vi "TrackStats2.vi"(0 "Last trial successful?":bool, 5 "Trial bin size":i32=100, 9 "Persistent\n Mode?":bool, 11 "Command":T1(ring)) -> (1 "Total incorrect":i32, 3 "Total correct":i32, 4 "# total trials":i32, 6 "Total % correct":dbl, 10 "Segment trials":i32, 12 "Experiment trials":i32, 13 "Experiment correct":i32, 14 "Experiment %":dbl, 15 "Segment Percentage":dbl)   [LabVIEW 2010]
panel:
  out "Experiment incorrect":i32
  out "Segment incorrect trials":i32
  out "Segment correct trials":i32
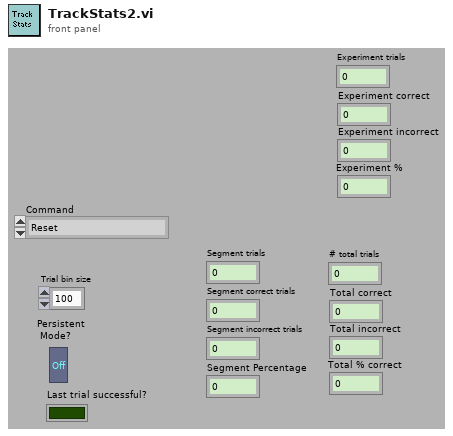
[diagram p1: front panel]
types:
  T1 = enum16{"Reset", "Increment", "Reset for exp", "Initialize"}
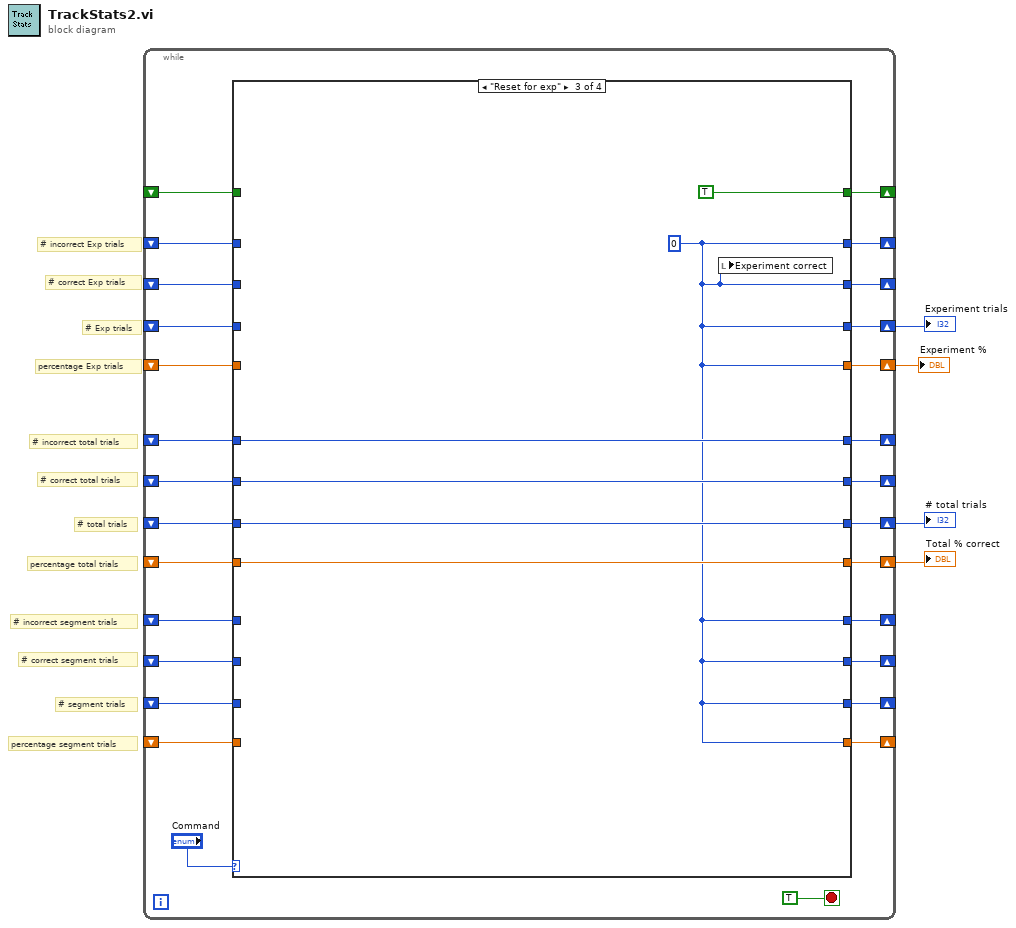
[diagram p0: block diagram]
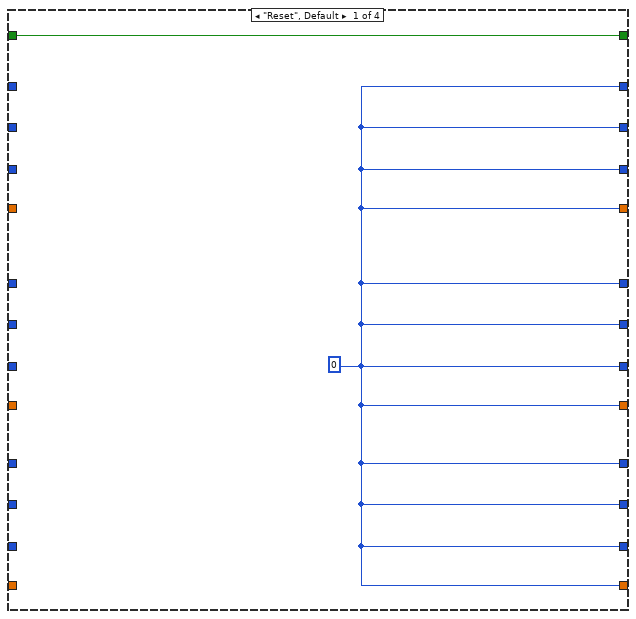
[diagram p2: hidden frame]
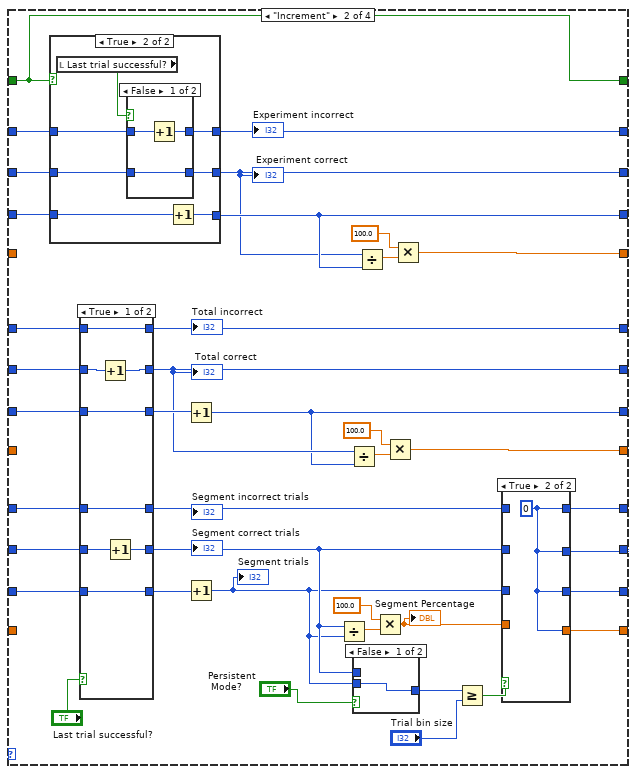
[diagram p3: hidden frame]
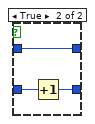
[diagram p5: hidden frame]
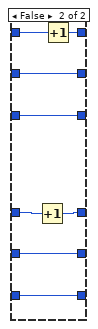
[diagram p8: hidden frame]
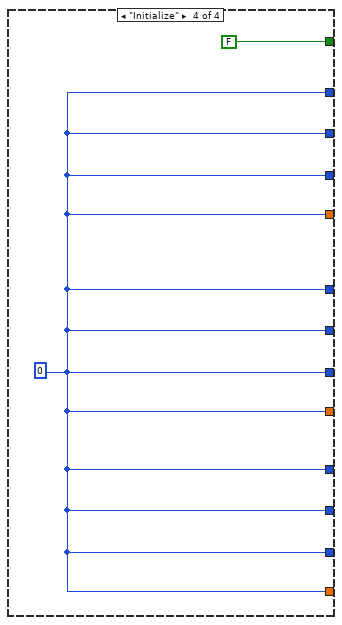
[diagram p9: hidden frame]
diagram:
  # "percentage Exp trials"
  # "# incorrect Exp trials"
  # "# correct Exp trials"
  # "# Exp trials"
  # "percentage total trials"
  # "# incorrect total trials"
  # "# correct total trials"
  # "# total trials"
  # "percentage segment trials"
  # "# incorrect segment trials"
  # "# correct segment trials"
  # "# segment trials"
  n1 = while {
    shift-right: [w17] -> _
    shift-left: _ -> [w30]
    shift-right: [w18] -> _
    shift-left: _ -> [w29]
    shift-right: [w19] -> _
    shift-left: _ -> [w28]
    shift-right: [w16] -> _
    shift-left: _ -> [w31]
    shift-right: [w23] -> w2
    shift-left: _ -> [w26]
    shift-right: [w22] -> _
    shift-left: _ -> [w25]
    shift-right: [w21] -> _
    shift-left: _ -> [w24]
    shift-right: [w20] -> w1
    shift-left: _ -> [w27]
    shift-right: [w11] -> w4
    shift-left: _ -> [w8]
    shift-right: [w12] -> _
    shift-left: _ -> [w9]
    shift-right: [w13] -> _
    shift-left: _ -> [w10]
    shift-right: [w14] -> w3
    shift-left: _ -> [w7]
    shift-right: [w6] -> _
    shift-left: _ -> [w5]
    stop <- TRUE stop-if-true
    n2 = case shown="\"Reset for exp\"" "Command" {
      tunnel: w31 -> [_ _ _ _]
      tunnel: w30 -> [_ w64 _ _]
      tunnel: w29 -> [_ w65 _ _]
      tunnel: w28 -> [_ w66 _ _]
      tunnel: w27 -> [_ _ w115 _]
      tunnel: w26 -> [_ w68 w116 _]
      tunnel: w25 -> [_ w69 w117 _]
      tunnel: w24 -> [_ w70 w118 _]
      tunnel: [w34 w61 w116 w119] -> w23
      tunnel: [w34 w62 w117 w119] -> w22
      tunnel: [w34 w63 w118 w119] -> w21
      tunnel: [w34 w57 w115 w119] -> w20
      tunnel: [w34 w52 w113 w119] -> w19
      tunnel: [w34 w53 w113 w119] -> w18
      tunnel: [w34 w54 w113 w119] -> w17
      tunnel: [w34 w55 w113 w119] -> w16
      tunnel: w7 -> [_ _ _ _]
      tunnel: w8 -> [_ w38 _ _]
      tunnel: w9 -> [_ w40 _ _]
      tunnel: w10 -> [_ w42 _ _]
      tunnel: [w34 w45 w113 w119] -> w11
      tunnel: [w34 w39 w113 w119] -> w12
      tunnel: [w34 w41 w113 w119] -> w13
      tunnel: [w34 w46 w113 w119] -> w14
      tunnel: [w33 w37 TRUE FALSE] -> w6
      tunnel: w5 -> [w33 w37 _ _]
      frame "Reset", Default {
        w34 = 0 ("Total correct")
      }
      frame "Increment" {
        n3 = case shown="True" w37 {
          tunnel: [w74 w83] -> w45
          tunnel: [w76 w79] -> w41
          tunnel: w42 -> [w76 w80]
          tunnel: [w75 w77] -> w39
          tunnel: w40 -> [w75 w78]
          tunnel: w38 -> [w74 w81]
          frame False {
          }
          frame True {
            n4 = local read "Last trial successful?"() -> (w82:bool)
            n5 = case shown="False" w82 {
              tunnel: [w84 w89] -> w79
              tunnel: w80 -> [w86 w89]
              tunnel: w78 -> [w85 w88]
              tunnel: [w85 w87] -> w77
              frame False {
                n6 = Increment(x=w86) -> (x+1=w84:i32)
              }
              frame True {
                n7 = Increment(x=w88) -> (x+1=w87:i32)
              }
            }
            n8 = Increment(x=w81) -> (x+1=w83:i32)
          }
        }
        "Experiment correct" <- w39
        "Experiment incorrect" <- w41
        n9 = case shown="True" "Last trial successful?" {
          tunnel: w70 -> [w102 w110]
          tunnel: w69 -> [w104 w112]
          tunnel: [w98 w112] -> w62
          tunnel: w68 -> [w103 w111]
          tunnel: [w103 w111] -> w67
          tunnel: [w102 w106] -> w63
          tunnel: [w101 w105] -> w51
          tunnel: w66 -> [w101 w109]
          tunnel: [w97 w108] -> w48
          tunnel: w65 -> [w100 w108]
          tunnel: [w99 w107] -> w60
          tunnel: w64 -> [w99 w107]
          frame True {
            n10 = Increment(x=w104) -> (x+1=w98:i32)
            n11 = Increment(x=w100) -> (x+1=w97:i32)
          }
          frame False {
            n12 = Increment(x=w109) -> (x+1=w105:i32)
            n13 = Increment(x=w110) -> (x+1=w106:i32)
          }
        }
        "Segment correct trials" <- w48
        "Segment incorrect trials" <- w51
        "Total correct" <- w62
        "Total incorrect" <- w63
        n14 = Increment(x=w67) -> (x+1=w61:i32)
        n15 = Increment(x=w60) -> (x+1=w36:i32)
        "Segment trials" <- w36
        n16 = Divide(x=w48, y=w36) -> (x/y=w58:dbl)
        n17 = Divide(x=w62, y=w61) -> (x/y=w73:dbl)
        n18 = case shown="False" "Persistent\n Mode?" {
          tunnel: w36 -> [w90 _]
          tunnel: w48 -> [_ w91]
          tunnel: [w90 w91] -> w47
          frame False {
          }
          frame True {
          }
        }
        n19 = Divide(x=w39, y=w45) -> (x/y=w43:dbl)
        n20 = Multiply(x=100.0, y=w58) -> (x*y=w35:dbl)
        "Segment Percentage" <- w35
        n21 = Multiply(x=100.0, y=w73) -> (x*y=w57:dbl)
        n22 = Multiply(x=100.0, y=w43) -> (x*y=w46:dbl)
        n23 = Greater Or Equal?(x=w47, y="Trial bin size") -> (x >= y?=w56:bool)
        n24 = case shown="True" w56 {
          tunnel: [w92 w96] -> w55
          tunnel: [w93 w96] -> w54
          tunnel: [w94 w96] -> w53
          tunnel: [w95 w96] -> w52
          tunnel: w51 -> [w95 _]
          tunnel: w48 -> [w94 _]
          tunnel: w36 -> [w93 _]
          tunnel: w35 -> [w92 _]
          frame False {
          }
          frame True {
            w96 = 0 ("Total correct")
          }
        }
      }
      frame "Reset for exp" {
        w113 = 0 ("Total correct")
        n25 = local write "Experiment correct"(w113) -> ()
      }
      frame "Initialize" {
        w119 = 0 ("Total correct")
      }
    }
  }
  "Experiment trials" <- w4
  "Experiment %" <- w3
  "# total trials" <- w2
  "Total % correct" <- w1
